vi "索引数据并插入.vi"(8 "error in (no error)":errorcluster, 10 "索引记录":timestamp format="%<%H:%M:%S\n%m/%d/%Y>T", 11 "table":string) -> (0 "error out":errorcluster, 3 "最新索引记录":timestamp)   [LabVIEW 2016, in "数据查询.lvlib"]
uses:
  <vilib>/Utility/sysdir.llb/System Directory Type.ctl
  <vilib>/addons/database/Auxilliary.llb/DB Tools Column Info.ctl
  <vilib>/addons/database/Auxilliary.llb/DB Tools DataTypes.ctl
  <vilib>/addons/database/Connection.llb/DB Tools Open Connec (String).vi
  <userlib>/_OpenG.lib/array/array.llb/Remove Duplicates from 1D Array (Variant)__ogtk.vi
  <userlib>/_OpenG.lib/array/array.llb/Sort 1D Array (I32)__ogtk.vi
  <vilib>/addons/database/_DB Variant To Data/Database Variant To Data.xnode
  <vilib>/Utility/VariantDataType/VariantType.lvlib
  <vilib>/addons/database/NI_Database_API.lvlib
panel:
  in  "表键":T1
  in  "data in":T2
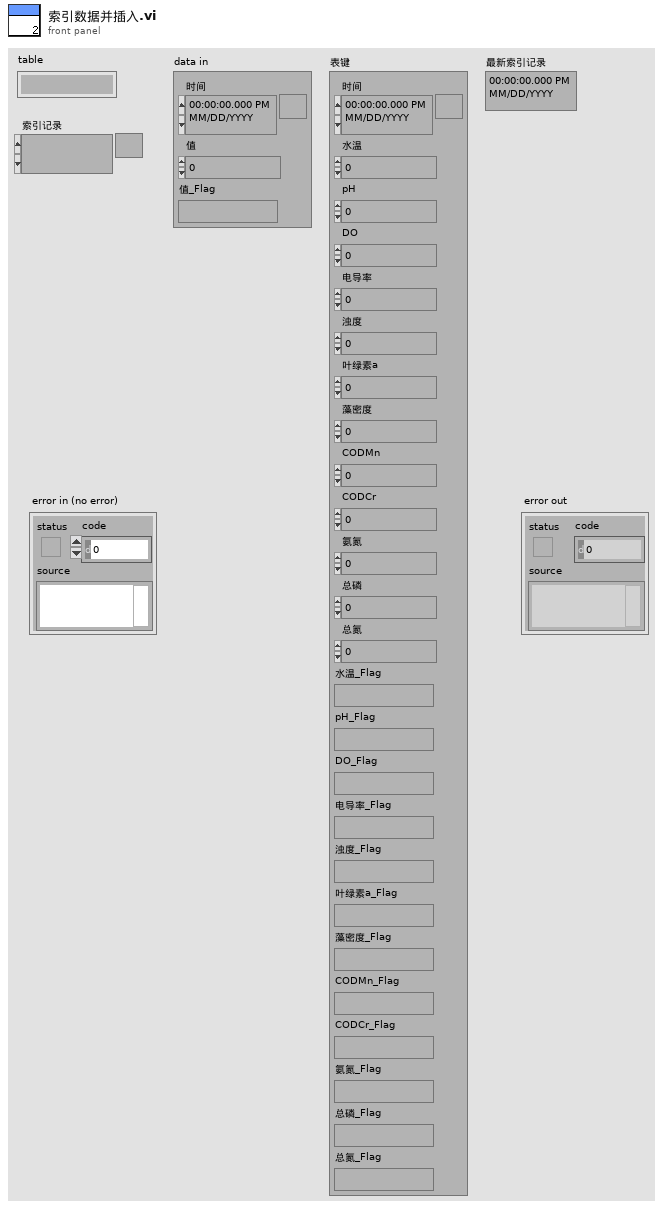
[diagram p1: front panel]
types:
  T1 = cluster{"时间":timestamp, "水温":sgl, "pH":sgl, "DO":sgl, "电导率":sgl, "浊度":sgl, "叶绿素a":sgl, "藻密度":sgl, "CODMn":sgl, "CODCr":sgl, "氨氮":sgl, "总磷":sgl, "总氮":sgl, "水温_Flag":string, "pH_Flag":string, "DO_Flag":string, "电导率_Flag":string, "浊度_Flag":string, "叶绿素a_Flag":string, "藻密度_Flag":string, "CODMn_Flag":string, "CODCr_Flag":string, "氨氮_Flag":string, "总磷_Flag":string, "总氮_Flag":string}
  T2 = cluster{"时间":timestamp, "值":sgl, "值_Flag":string}
  T3 = typedef "System Directory Type.ctl" = i32
  T4 = cluster{"时间":timestamp, "值":sgl, "值_Flag":string}[]
  T5 = typedef "NI_Database_API.lvlib/Conn ObjectReference.ctl" = refnum<k1>
  T6 = typedef "LVDateTimeRec.ctl" = cluster{"秒数的小数部分":dbl, "秒":i32, "分":i32, "时":i32, "日":i32, "月":i32, "年":i32, "天数（周）":i32, "天数（年）":i32, "DST":i32}
  T7 = typedef "NI_Database_API.lvlib/DB Tools Column Info.ctl" = cluster{"column name":string, "data type":T8, "size":i32, "allow null?":bool}
  T8 = typedef "NI_Database_API.lvlib/DB Tools DataTypes.ctl" = enum16{"String", "Long (I32)", "Single (SGL)", "Double (DBL)", "Date/Time", "Binary"}
  T9 = typedef "VariantType.lvlib/Type.ctl" = enum8{"Invalid Type", "Void", "I8", "I16", "I32", "I64", "U8", "U16", "U32", "U64", "Single Float", "Double Float", "Extended Float", "Single Complex", "Double Complex", "Extended Complex", "Enum U8", "Enum U16", "Enum U32", "Enum U64", "Single Float With Unit", "Double Float With Unit", "Extended Float With Unit", "Single Complex with Unit", "Double Complex with Unit", "Extended Complex with Unit", "Boolean", "String", "Path", "Picture", "Tag", "Array", "Cluster", "Variant", "LV Variant", "Waveform", "Timestamp", "Digital Waveform", "Digital Data", "ExpressData", "Refnum", "External Data", "VI", "Poly VI", "LabVIEW Class Instance", "Fixed Point"}
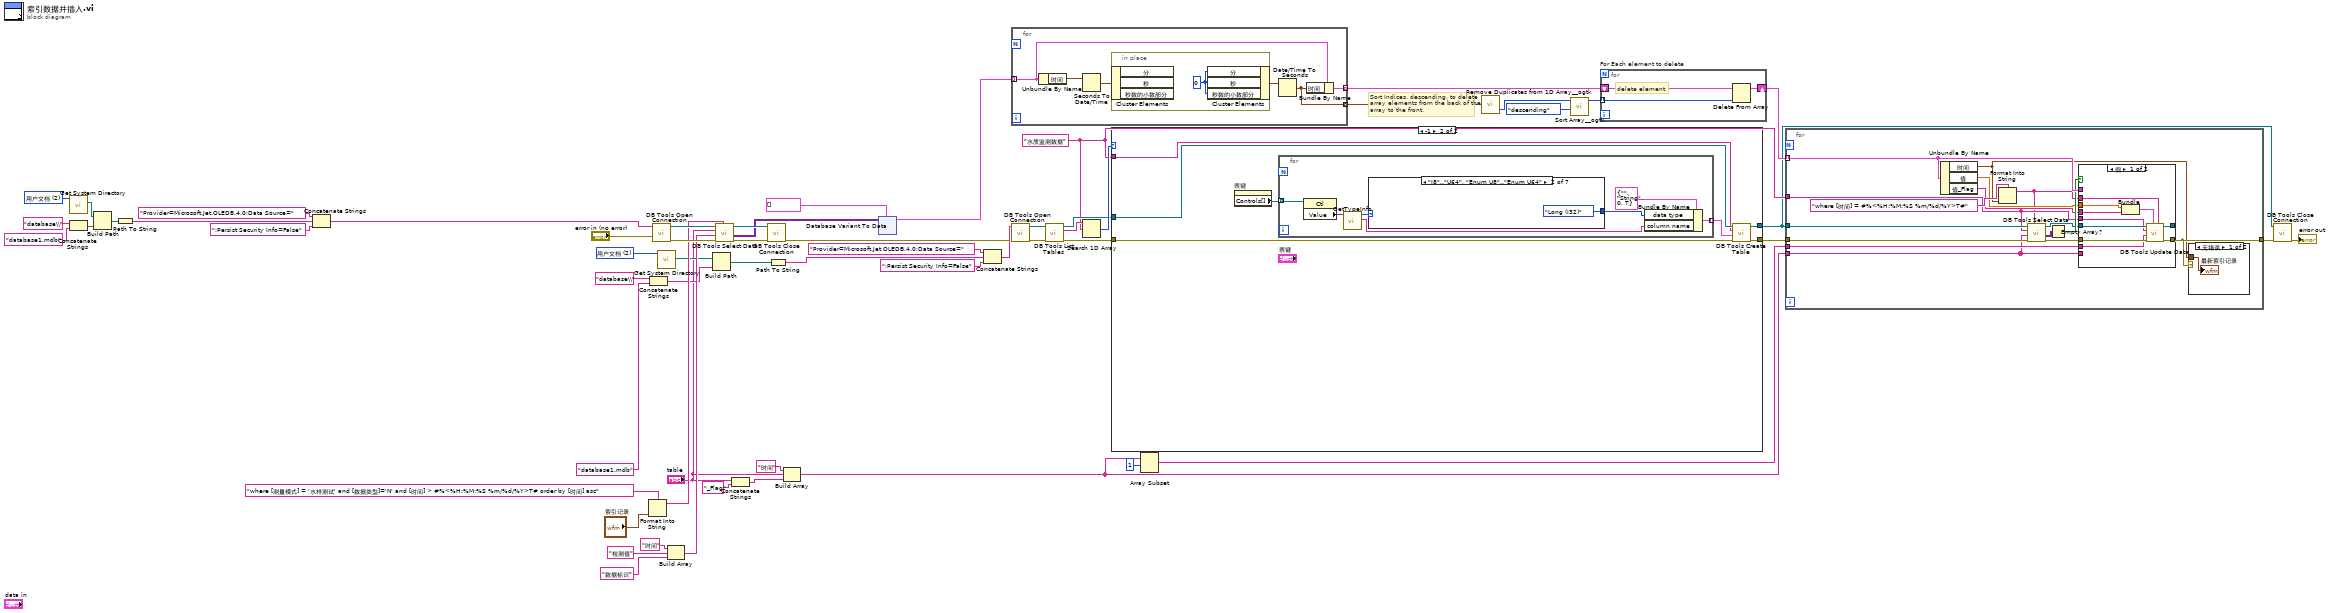
[diagram p0: block diagram]
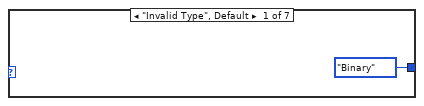
[diagram p3: hidden frame]
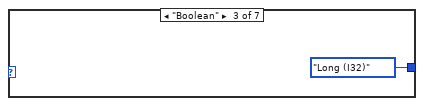
[diagram p4: hidden frame]
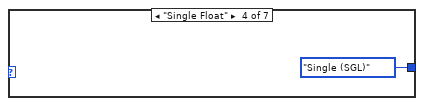
[diagram p5: hidden frame]
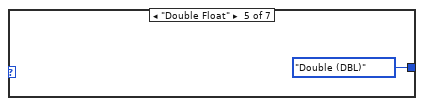
[diagram p6: hidden frame]
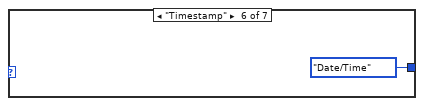
[diagram p7: hidden frame]
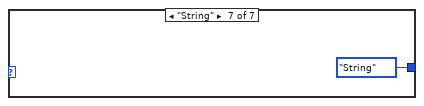
[diagram p8: hidden frame]
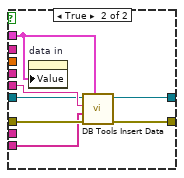
[diagram p10: hidden frame]
diagram:
  w11 = "水质监测数据" ("table")
  w21 = T3 2 items=["用户目录"=0, "用户桌面"=1, "用户文档"=2, "用户应用程序数据"=3, "用户设置"=4, "用户临时目录"=5, "公共文档"=6, "公共应用程序数据"=7, "公共设置"=8, "公共缓存"=13, "系统核心库"=9, "系统安装库"=10, "应用程序文件"=11, "启动盘根目录"=12] ("system directory type")
  w43 = T3 2 items=["用户目录"=0, "用户桌面"=1, "用户文档"=2, "用户应用程序数据"=3, "用户设置"=4, "用户临时目录"=5, "公共文档"=6, "公共应用程序数据"=7, "公共设置"=8, "公共缓存"=13, "系统核心库"=9, "系统安装库"=10, "应用程序文件"=11, "启动盘根目录"=12] ("system directory type")
  # "Sort Indices, descending, to delete array elements from the back of the array to the front."
  n1 = call <vilib>:"Get System Directory.vi"("system directory type"=w43) -> ("system directory"=w41:path)  [unwired: 10 in]
  n2 = Concatenate Strings("database\\" ("condition"), "database1.mdb" ("字符串")) -> (w35:string)
  n3 = Build Path(base path=w41, name or relative path=w35) -> (appended path=w40:path)
  n4 = Path To String(path=w40) -> (string=w39:string)
  n5 = Concatenate Strings("Provider=Microsoft.Jet.OLEDB.4.0;Data Source=" ("condition"), w39, ";Persist Security Info=False" ("condition")) -> (w37:string)
  n6 = Format Into String(format string="where [测量模式] = '水样测试' and [数据类型]='N' and [时间] > #%<%H:%M:%S %m/%d/%Y>T# order by [时间] asc" ("condition"), "索引记录") -> (resulting string=w32:string)  [unwired: 2 in, 1 out]
  n7 = Concatenate Strings("database\\" ("condition"), "database1.mdb" ("字符串")) -> (w29:string)
  n8 = call-poly <vilib>:"DB Tools Open Connection.vi"("error in (no error)"="error in (no error)", "connection information"=w37) -> ("error out"=w45:errorcluster, "connection reference"=w47:T5)  [unwired: 6 in]
  n9 = call <vilib>:"Get System Directory.vi"("system directory type"=w21) -> ("system directory"=w23:path)  [unwired: 10 in]
  n10 = Build Array("时间", "检测值" ("元素"), "数据标识" ("字符串")) -> (w31:string[])
  n11 = Build Path(base path=w23, name or relative path=w29) -> (appended path=w24:path)
  n12 = call <vilib>:"DB Tools Select Data.vi"("condition"=w32, "error in (no error)"=w45, "columns"=w31, "table"="table", "connection reference"=w47) -> ("error out"=w44:errorcluster, "data"=w33:variant[][], "connection reference out"=w46:T5)  [unwired: 1 in]
  n13 = Concatenate Strings("table", "_Flag") -> (w6:string)
  n14 = call <vilib>:"DB Tools Close Connection.vi"("error in (no error)"=w44, "connection reference"=w46) -> ("error out"=w19:errorcluster)  [unwired: 5 in]
  n15 = Path To String(path=w24) -> (string=w25:string)
  n16 = Build Array("时间", "table", w6) -> (w5:string[])
  n17 = xnode "Database Variant To Data"("database variant"=w33, "type"=T4 []) -> ("data"=w55:T4)  [unwired: 1 in, 1 out]
  n18 = Concatenate Strings("Provider=Microsoft.Jet.OLEDB.4.0;Data Source=" ("condition"), w25, ";Persist Security Info=False" ("condition")) -> (w27:string)
  n19 = for {
    tunnel: [w66] -> w52 mode=indexing
    tunnel: [w62] -> w56 mode=indexing
    tunnel: w55 -> [w61] mode=indexing
    n20 = Unbundle By Name(w61) -> ("时间"=w65:timestamp)
    n21 = Seconds To Date/Time(time stamp (now)=w65) -> (date time rec=w64:T6)  [unwired: 1 in]
    n22 = in-place {
      w67 = 0 ("分")
      n23 = in-place-cluster #1(w64) -> ()  [unwired: 3 out]
      n24 = in-place-cluster #1("分"=w67, "秒"=w67, "秒数的小数部分"=w67) -> (w63:T6)
    }
    n25 = Date/Time To Seconds(2:w63) -> (0:w62:timestamp)  [unwired: 1 in]
    n26 = Bundle By Name(cluster=w61, "时间"=w62) -> (w66:T2)
  }
  n27 = call-poly <vilib>:"DB Tools Open Connection.vi"("error in (no error)"=w19, "connection information"=w27) -> ("error out"=w17:errorcluster, "connection reference"=w18:T5)  [unwired: 6 in]
  n28 = call <vilib>:"DB Tools List Tables.vi"("error in (no error)"=w17, "connection reference"=w18) -> ("error out"=w13:errorcluster, "tables"=w16:string[], "connection reference out"=w14:T5)  [unwired: 3 in]
  n29 = Search 1D Array(1D array=w16, element=w11) -> (index of element=w15:i32)  [unwired: 1 in]
  n30 = case shown="-1" w15 {
    tunnel: w14 -> [w69 w74]
    tunnel: w13 -> [w68 w72]
    tunnel: [w69 w71] -> w10
    tunnel: [w68 w70] -> w12
    tunnel: w11 -> [_ w73]
    frame 0, Default {
    }
    frame -1 {
      n31 = property on="表键" class="Clust (严格)"() -> ("Controls[]"=w75:refnum<vi>[])  [unwired: 2 in, 2 out]
      n32 = for {
        tunnel: w75 -> [w83] mode=indexing
        tunnel: [w79] -> w76 mode=indexing
        n33 = property class="Ctl"(reference=w83) -> ("Value"=w78:variant)  [unwired: 1 in, 2 out]
        n34 = call <vilib>:"GetTypeInfo.vi"("Variant"=w78) -> ("Name"=w77:string, "Type Enum"=w81:T9)  [unwired: 6 in, 3 out]
        n35 = case shown="\"I8\"..\"U64\", \"Enum U8\"..\"Enum U64\"" w81 {
          tunnel: [DB_Tools_DataTypes."Binary" ("data type") DB_Tools_DataTypes."Long (I32)" ("data type") DB_Tools_DataTypes."Long (I32)" ("data type") DB_Tools_DataTypes."Single (SGL)" ("data type") DB_Tools_DataTypes."Double (DBL)" ("data type") DB_Tools_DataTypes."Date/Time" ("data type") DB_Tools_DataTypes."String" ("data type")] -> w80
          frame "Invalid Type", Default {
          }
          frame "I8".."U64", "Enum U8".."Enum U64" {
          }
          frame "Boolean" {
          }
          frame "Single Float" {
          }
          frame "Double Float" {
          }
          frame "Timestamp" {
          }
          frame "String" {
          }
        }
        n36 = Bundle By Name(cluster=T7 {"column name"="", "data type"=enum."String", "size"=0, "allow null?"=TRUE} ("column information"), "data type"=w80, "column name"=w77) -> (w79:T7)
      }
      n37 = call <vilib>:"DB Tools Create Table.vi"("error in (no error)"=w72, "column information"=w76, "table"=w73, "connection reference"=w74) -> ("error out"=w70:errorcluster, "connection reference out"=w71:T5)  [unwired: 4 in]
    }
  }
  n38 = Array Subset(array=w5, index=1 ("索引")) -> (w3:string[])  [unwired: 1 in]
  n39 = call-poly <userlib>:"Remove Duplicates from 1D Array__ogtk.vi"("Input Array"=w56) -> ("indices of removed elements"=w51:i32[])  [unwired: 1 out]
  n40 = call-poly <userlib>:"Sort Array__ogtk.vi"("Order"=enum16{"ascending", "descending"}."descending", "Array in"=w51) -> ("Sorted Array out"=w53:i32[])  [unwired: 8 in, 1 out]
  n41 = for "For Each element to delete" {
    tunnel: w53 -> [w93] mode=indexing
    shift-right: [w92] -> w50
    shift-left: w52 -> [w91]
    # "delete element"
    n42 = Delete From Array(array=w91, index=w93) -> (array with subset deleted=w92:T4)  [unwired: 1 in, 1 out]
  }
  n43 = for {
    tunnel: w50 -> [w108] mode=indexing
    tunnel: w10 -> [w106]
    tunnel: w12 -> [w105]
    tunnel: [w95] -> w20
    tunnel: w11 -> [w102]
    tunnel: w5 -> [w96]
    tunnel: w3 -> [w98]
    n44 = Unbundle By Name(w108) -> ("时间"=w94:timestamp, "值"=w100:sgl, "值_Flag"=w99:string)
    n45 = Format Into String(format string="where [时间] = #%<%H:%M:%S %m/%d/%Y>T#" ("condition"), w94) -> (resulting string=w97:string)  [unwired: 2 in, 1 out]
    n46 = call <vilib>:"DB Tools Select Data.vi"("condition"=w97, "error in (no error)"=w105, "columns"=w96, "table"=w102, "connection reference"=w106) -> ("error out"=w103:errorcluster, "data"=w101:variant[][], "connection reference out"=w104:T5)  [unwired: 1 in]
    n47 = Empty Array?(array=w101) -> (empty?=w107:bool)
    n48 = case shown="假" w107 {
      tunnel: w108 -> [_ w125]
      tunnel: w102 -> [w116 w127]
      tunnel: w104 -> [w120 w126]
      tunnel: w103 -> [w119 w124]
      tunnel: [w117 w122] -> w95
      tunnel: [w118 w123] -> _
      tunnel: w100 -> [w114 _]
      tunnel: w99 -> [w115 _]
      tunnel: w98 -> [w112 _]
      tunnel: w97 -> [w111 _]
      tunnel: w96 -> [_ w121]
      frame False {
        n49 = Bundle("值"=w114, "值_Flag"=w115) -> (w113:cluster{"值":sgl, "值_Flag":string})  [unwired: 1 in]
        n50 = call <vilib>:"DB Tools Update Data.vi"("condition"=w111, "data"=w113, "error in (no error)"=w119, "columns"=w112, "table"=w116, "connection reference"=w120) -> ("error out"=w117:errorcluster, "connection reference out"=w118:T5)  [unwired: 4 in]
      }
      frame True {
        n51 = property on="data in" class="Clust (严格)"("Value"=w125) -> ()  [unwired: 2 in, 2 out]
        n52 = call <vilib>:"DB Tools Insert Data.vi"("data"=w125, "error in (no error)"=w124, "columns"=w121, "table"=w127, "connection reference"=w126) -> ("error out"=w122:errorcluster, "connection reference out"=w123:T5)  [unwired: 5 in]
      }
    }
    n53 = case shown="无错误" w95 {
      tunnel: w94 -> [w110 _]
      frame No Error {
        "最新索引记录" <- w110
      }
      frame Error {
      }
    }
  }
  n54 = call <vilib>:"DB Tools Close Connection.vi"("error in (no error)"=w20, "connection reference"=w10) -> ("error out"=→"error out":errorcluster)  [unwired: 5 in]
